vi "convert-direction-enum-to-cluster-of-booleans.vi"(11 "gamepad direction":T1) -> (3 "Direction":T2)   [LabVIEW 2020, in "GUI.lvlib"]
uses:
  GUI.lvlib
  Shared Ressources/gamepad-direction-enum.ctl
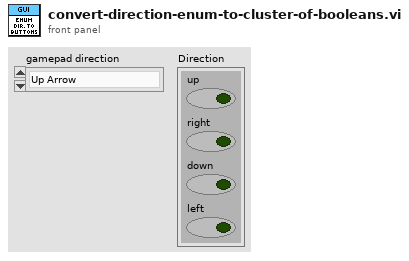
[diagram p1: front panel]
types:
  T1 = typedef "gamepad-direction-enum.ctl" = enum16{"Up Arrow", "Right Arrow", "Down Arrow", "Left Arrow"}
  T2 = cluster{"up":bool, "right":bool, "down":bool, "left":bool}
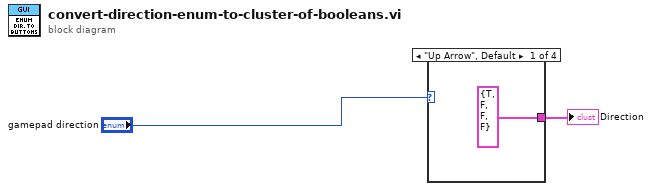
[diagram p0: block diagram]
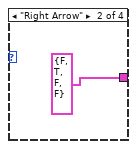
[diagram p2: hidden frame]
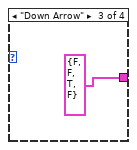
[diagram p3: hidden frame]
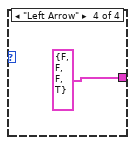
[diagram p4: hidden frame]
diagram:
  n1 = case shown="\"Up Arrow\", Default" "gamepad direction" {
    tunnel: [T2 {"up"=TRUE, "right"=FALSE, "down"=FALSE, "left"=FALSE} ("Direction") T2 {"up"=FALSE, "right"=TRUE, "down"=FALSE, "left"=FALSE} ("Direction") T2 {"up"=FALSE, "right"=FALSE, "down"=TRUE, "left"=FALSE} ("Direction") T2 {"up"=FALSE, "right"=FALSE, "down"=FALSE, "left"=TRUE} ("Direction")] -> w2
    frame "Up Arrow", Default {
    }
    frame "Right Arrow" {
    }
    frame "Down Arrow" {
    }
    frame "Left Arrow" {
    }
  }
  "Direction" <- w2
